vi "Parse String Lines.vi"(0 "multi-line string":string, 1 "delimiter":T1(ring)) -> (5 "lines":string[](array[string]))   [LabVIEW 2016]
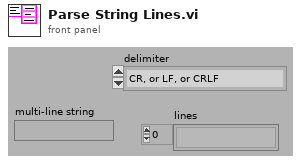
[diagram p1: front panel]
types:
  T1 = enum16{"CR, or LF, or CRLF", "CR (Mac)", "LF (Unix)", "CRLF (Windows)", "From OS"}
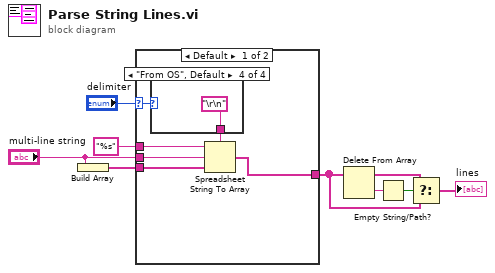
[diagram p0: block diagram]
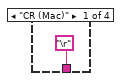
[diagram p2: hidden frame]
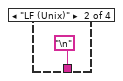
[diagram p3: hidden frame]
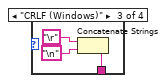
[diagram p4: hidden frame]
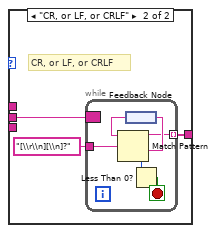
[diagram p5: hidden frame]
diagram:
  n1 = Build Array("multi-line string") -> (w4:string[])
  n2 = case shown="Default" "delimiter" {
    selector: "delimiter" -> [w12 _]
    tunnel: [w11 w23] -> w5
    tunnel: w4 -> [w15 _]
    tunnel: "multi-line string" -> [w14 w22]
    tunnel: "%s" ("format string") -> [w13 _]
    frame Default {
      n3 = case shown="\"From OS\", Default" w12 {
        tunnel: ["\r" "\n" w20 "\r\n"] -> w10
        frame "CR (Mac)" {
        }
        frame "LF (Unix)" {
        }
        frame "CRLF (Windows)" {
          n4 = Concatenate Strings("\r", "\n") -> (w20:string)
        }
        frame "From OS", Default {
        }
      }
      n5 = Spreadsheet String To Array(delimiter (Tab)=w10, format string=w13, spreadsheet string=w14, array type (2D Dbl)=w15) -> (array=w11:string[])
    }
    frame "CR, or LF, or CRLF" {
      # "CR, or LF, or CRLF"
      n6 = while {
        tunnel: "[\\r\\n][\\n]?" -> [w29]
        tunnel: [w27] -> w23 mode=indexing
        border: w22 -> [_]
        stop <- w26 stop-if-true
        n7 = feedback #1() -> (w30:string)
        n8 = Match Pattern(string=w30, regular expression=w29) -> (before substring=w27:string, after substring=w28:string, offset past match=w25:i32)  [unwired: 1 in, 1 out]
        n9 = feedback-in #1(w28) -> ()
        n10 = Less Than 0?(x=w25) -> (x < 0?=w26:bool)
      }
    }
  }
  n11 = Delete From Array(array=w5) -> (deleted portion=w9:string, array with subset deleted=w7:string[])  [unwired: 2 in]
  n12 = Empty String/Path?(string/path=w9) -> (empty?=w8:bool)
  n13 = Select(t=w7, s=w8, f=w5) -> (s? t:f=→"lines":string[])
